vi "OpenByRefnumAndRunBD.vi"(0 "VI refnum":refnum<vi>, 1 "Input data timeout":i32=-1 caption="Input data timeout (-1) [ms]" min=-1, 5 "Wait until VI done?":bool caption="Wait until VI done? (F)", 7 "Auto dispose VI refnum?":bool=TRUE caption="Auto dispose VI refnum? (T)", 9 "Reentrancy mode":T2=enum."Auto" caption="Reentrancy mode (Auto)", 11 "Error in":errorcluster caption="Error in (no error)", 12 "Input data names":string[](array[string]) caption="Input data names (none)", 13 "Input data values":variant[](array[variant]) caption="Input data values (none)") -> (2 "Input data timed out?":bool, 3 "VI refnum opened?":bool, 4 "VI refnum out":refnum<vi>, 6 "VI running?":bool, 8 "Last execution state":T1(ring), 10 "VI refnum opened as reentrant?":bool, 14 "Input data delivered?":bool, 15 "Error out":errorcluster)   [LabVIEW 2017, in "VILauncher.lvlib"]
doc: "Opens a reference to a dynamic VI either specified by path (<B>VI path</B>) or by reference (<B>VI refnum</B>), runs the dynamic VI, and returns the reference to it in <B>VI refnum out</B>.\n\nThis function will wait until the dynamic VI is done if <B>Wait until VI done?</B> is True (default is False), and it will auto dispose the dynamic VI reference (hand it over to the running dynamic VI) if <B>Auto dispose VI refnum?</B> is True. Note that if this function fails to run the dynamic VI, it will close the opened VI reference itself, in which case <B>VI refnum opened?</B> will be False and <B>VI refnum out</B> will be invalid.\n\nUse the optional <B>Reentrancy mode</B> input to specify whether the dynamic VI should be opened as a reentrant or a non-reentrant instance. Set this to Auto (default) to first try as reentrant, and if that fails, as non-reentrant. The <B>VI refnum opened as reentrant?</B> output will reflect the eventual instantiation mode.\n\nThe <B>VI running?</B> output will only be True if the dynamic VI's <B>Last execution state</B> is \"Run top level\". <B>VI running?</B> can be False even if the dynamic VI ran successfully - it might just have finished before this VI finished.\n\nOptionally you can send input data to the dynamic VI when running it using one of two modes; Right click this VI and use the Select Type menu to choose input data transfer mode:\n\nInput data via front panel\n-------------------------------\nSet data on the front panel of the dynamic VI before running it by wiring <B>Control names</B> and <B>Control values</B>. <B>Control values set?</B> will be True only if all <B>Control names</B> were valid.\n\nInput data via block diagram\n----------------------------------\nTransmit data to the dynamic VI after it has started by wiring <B>Input data names</B> and <B>Input data values</B>. If you use this mode the dynamic VI must use the WaitForInputData function to read the input data on the block diagram. The read in the dynamic VI must be finished before <B>Input data timeout</B> runs out. Set this timeout value to -1 (default) to wait indefinitely. If timeout does occur, <B>Input data timed out?</B> will be True. <B>Input data delivered?</B> will be True only if input data was in fact transmitted to the dynamic VI without any errors.\n\n<B>NOTE 1:</B> When using the 'Input data via block diagram' mode the dynamic VI must use the WaitForInputData function even if you send zero input data. To avoid this requirement for the dynamic VI when not passing any input data, please use the 'Input data via front panel' mode in this case.\n\n<B>NOTE 2:</B> The dynamic VI must have its front panel available at runtime for this function to work. The simplest way to ensure this, which also works in a built application without additional steps to be taken, is by enabling \"Show front panel when called\" in the \"Window Appearance\" section of the dynamic VI Properties.\n\nThis VI is reentrant, and it will only run if there is no error on <B>Error in</B>.\n\nSteen Schmidt\nGPower\n2/1 2013"
uses:
  VILauncher.lvlib
  Typedefs/ReentrancyMode.ctl
panel:
  # "Copyright © 2013\nGPower\nSee enclosed license file for terms and conditions"
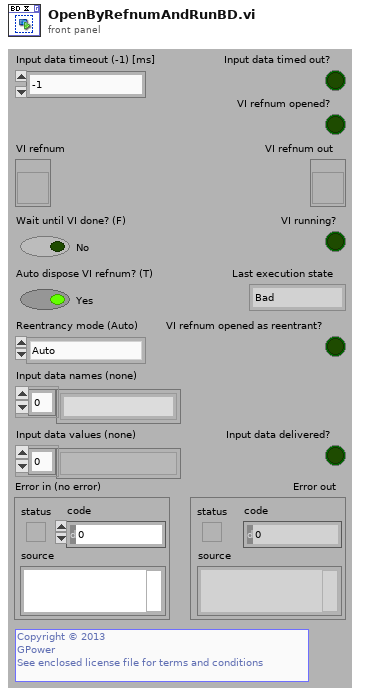
[diagram p1: front panel]
types:
  T1 = enum32{"Bad", "Idle", "Run top level", "Running"}
  T2 = typedef "VILauncher.lvlib/ReentrancyMode.ctl" = enum16{"Reentrant", "Non-reentrant", "Auto"}
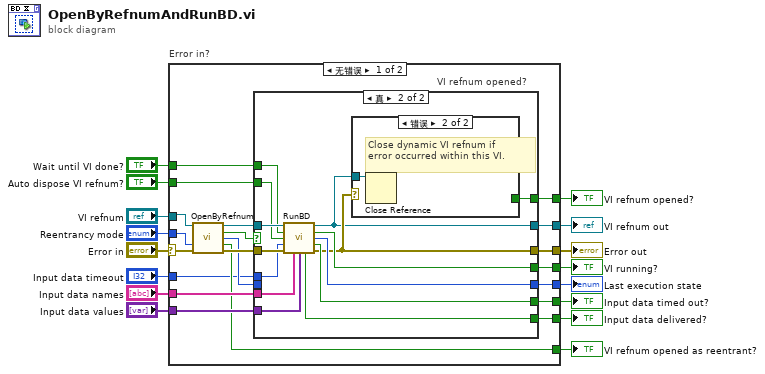
[diagram p0: block diagram]
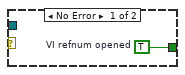
[diagram p3: hidden frame]
diagram:
  n1 = case "Error in?" shown="无错误" "Error in" {
    selector: "Error in" -> [w34 w56]
    tunnel: [w29 w56] -> w15
    tunnel: "Input data names" -> [w36 _]
    tunnel: "Input data values" -> [w35 _]
    tunnel: [w28 _] -> w12
    tunnel: "VI refnum" -> [w17 _]
    tunnel: "Reentrancy mode" -> [w32 _]
    tunnel: [w26 _] -> w10
    tunnel: "Auto dispose VI refnum?" -> [w25 _]
    tunnel: "Input data timeout" -> [w24 _]
    tunnel: [w23 _] -> w7
    tunnel: [w22 _] -> w6
    tunnel: [w21 _] -> w5
    tunnel: "Wait until VI done?" -> [w20 _]
    tunnel: [w19 _] -> w3
    tunnel: [w18 _] -> w2
    frame No Error {
      n2 = call "OpenByRefnum.vi"("VI refnum"=w17, "Reentrancy mode"=w32, "Error in"=w34) -> ("VI refnum out"=w30:refnum<vi>, "VI refnum opened?"=w31:bool, "Last execution state"=w27:T1, "VI refnum opened as reentrant?"=w26:bool, "Error out"=w33:errorcluster)  [unwired: 8 in]
      n3 = case "VI refnum opened?" shown="真" w31 {
        tunnel: w36 -> [_ w49]
        tunnel: w35 -> [_ w48]
        tunnel: w33 -> [w38 w53]
        tunnel: w30 -> [w39 w52]
        tunnel: [w38 w42] -> w29
        tunnel: [w39 w41] -> w28
        tunnel: w27 -> [w37 _]
        tunnel: w25 -> [_ w50]
        tunnel: w24 -> [_ w47]
        tunnel: [_ w43] -> w23
        tunnel: [_ w44] -> w22
        tunnel: [w37 w45] -> w21
        tunnel: w20 -> [_ w51]
        tunnel: [_ w46] -> w19
        tunnel: [_ w40] -> w18
        frame False {
        }
        frame True {
          n4 = call "RunBD.vi"("VI refnum in"=w52, "Wait until VI done?"=w51, "Auto dispose VI refnum?"=w50, "Input data timeout"=w47, "Error in"=w53, "Input data names"=w49, "Input data values"=w48) -> ("VI refnum out"=w41:refnum<vi>, "VI running?"=w44:bool, "Last execution state"=w45:T1, "Input data timed out?"=w43:bool, "Input data delivered?"=w46:bool, "Error out"=w42:errorcluster)  [unwired: 3 in]
          n5 = case shown="错误" w42 {
            tunnel: w41 -> [_ w55]
            tunnel: [w54 _] -> w40
            frame No Error {
              w54 = TRUE  # VI refnum opened
            }
            frame Error {
              # "Close dynamic VI refnum if\nerror occurred within this VI."
              n6 = Close Reference(reference=w55) -> ()  [unwired: 1 in, 1 out]
            }
          }
        }
      }
    }
    frame Error {
    }
  }
  "Error out" <- w15
  "VI refnum out" <- w12
  "VI running?" <- w6
  "VI refnum opened as reentrant?" <- w10
  "Last execution state" <- w5
  "Input data timed out?" <- w7
  "Input data delivered?" <- w3
  "VI refnum opened?" <- w2
